vi "Cubic m3 per voxel.vi"(2 "Scale ( µm )":ext) -> (7 "Numeric":ext, 9 "m3/vox":ext)   [LabVIEW 2020]
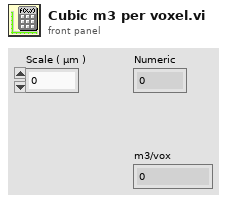
[diagram p1: front panel]
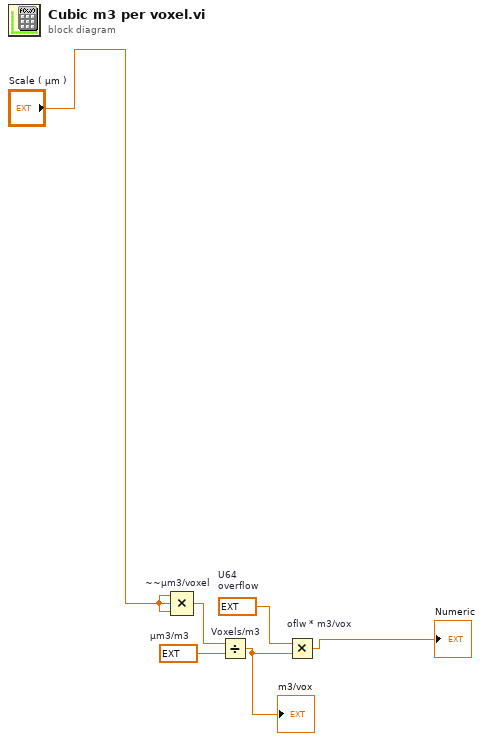
[diagram p0: block diagram]
diagram:
  w4 = ext 1e+18  # µm3/m3
  w2 = ext 2e+19  # U64 overflow
  n1 = Compound Arithmetic op=MULTIPLY "~~µm3/voxel"("Scale ( µm )", "Scale ( µm )", "Scale ( µm )") -> (w3:ext)
  n2 = Divide "Voxels/m3"(x=w3, y=w4) -> (x/y=w5:ext)
  "m3/vox" <- w5
  n3 = Multiply "oflw * m3/vox"(x=w2, y=w5) -> (x*y=→"Numeric":ext)
